vi "Downloader.vi"(8 "error in":errorcluster, 9 "Target Path":string="c:\\temp\\", 10 "Source URL":string) -> (0 "error out":errorcluster)   [LabVIEW 2016]
panel:
  out "Progress":u8(slide) scale=0.0..100.0
  in  "Files":string[](array[string])=["050523_fg_lv_cont_des.gif", "tagline.gif", "logo.gif"]
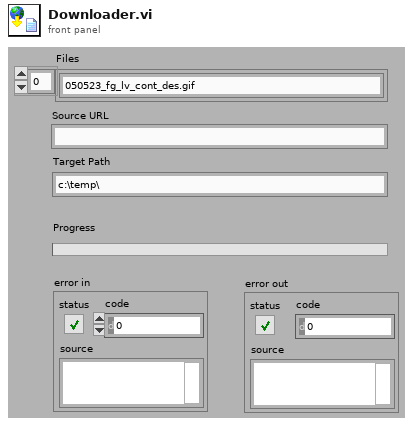
[diagram p1: front panel]
types:
  T1 = enum16{"open", "open or create", "create or replace", "create", "open (read only)"}
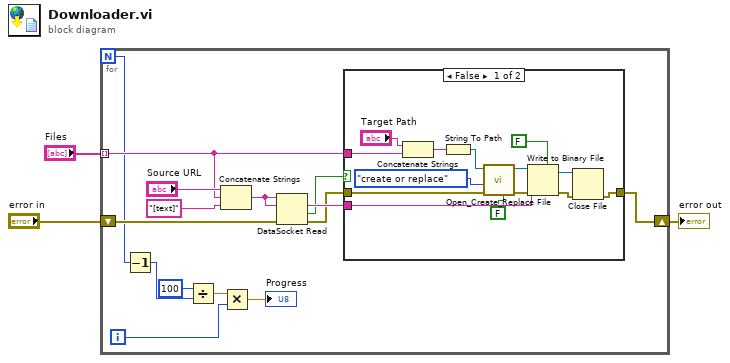
[diagram p0: block diagram]
diagram:
  n1 = for {
    N -> [w5]
    tunnel: "Files" -> [w14] mode=indexing
    shift-right: [w12] -> w1
    shift-left: "error in" -> [w11]
    i -> [w6]
    n2 = Decrement(x=w5) -> (x-1=w4:i32)
    n3 = Divide(x=100 ("y"), y=w4) -> (x/y=w9:dbl)
    n4 = Concatenate Strings("Source URL", w14, "[text]" ("string")) -> (w18:string)
    n5 = Multiply(x=w9, y=w6) -> (x*y=→"Progress":dbl)
    n6 = DataSocket Read(8:w11, 10:w18, 11:w18) -> (0:w13:errorcluster, 1:w10:bool, 2:w15:string)  [unwired: 2 in, 4 out]
    n7 = case shown="False" w10 {
      tunnel: w15 -> [w32 _]
      tunnel: w14 -> [w22 _]
      tunnel: w13 -> [w21 w33]
      tunnel: [w20 w33] -> w12
      frame False {
        n8 = Concatenate Strings("Target Path", w22) -> (w23:string)
        n9 = String To Path(string=w23) -> (path=w25:path)
        n10 = call <vilib>:"Open_Create_Replace File.vi"("advisory dialog? (display:T)"=FALSE, "error in (no error)"=w21, "function (open:0)"=T1."create or replace", "file path"=w25) -> ("error out"=w27:errorcluster, "refnum"=w31:refnum<file>)  [unwired: 4 in, 2 out]
        n11 = Write to Binary File(file (use dialog)=w31, data=w32, error in=w27, 5:FALSE ("prepend array or string size? (T)")) -> (refnum out=w30:refnum<file>, error out=w29:errorcluster)  [unwired: 2 in, 1 out]
        n12 = Close File(refnum=w30, error in=w29) -> (error out=w20:errorcluster)  [unwired: 1 out]
      }
      frame True {
      }
    }
  }
  "error out" <- w1
